vi "foobar.vi"(8 "error in (no error)":errorcluster, 11 "Model in":refnum<class "Model.lvclass">) -> (0 "error out":errorcluster, 3 "Model out":refnum<class "Model.lvclass">)   [LabVIEW 2016, in "Model.lvclass"]
uses:
  Model.lvclass
  Model.lvclass/Model.ctl
  ILCCommunications/ILCCommunications.lvclass
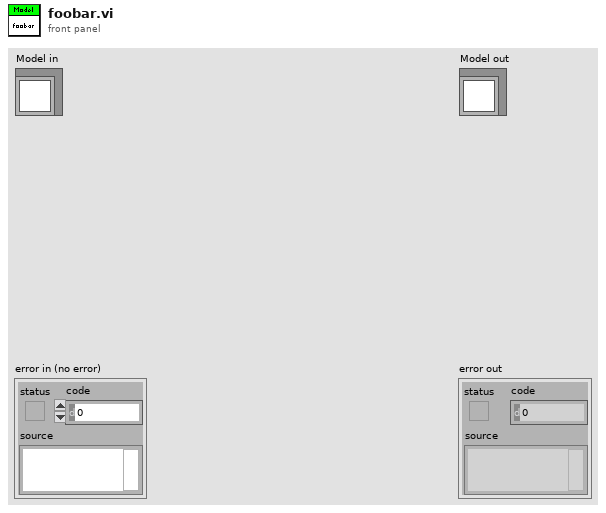
[diagram p1: front panel]
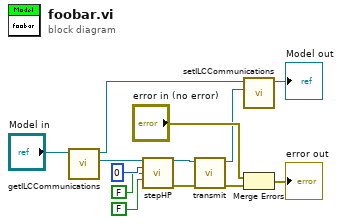
[diagram p0: block diagram]
diagram:
  n1 = call "getILCCommunications.vi"("Model in"="Model in") -> ("ILCCommunications"=w10:refnum<class "ILCCommunications.lvclass">, "Model out"=w4:refnum<class "Model.lvclass">)  [unwired: 9 in]
  n2 = call "stepHP.vi"("ILCCommunications in"=w10, "HPIndex"=0, "WaitForTrigger"=FALSE, "TriggerIRQ"=FALSE) -> ("ILCCommunications out"=w6:refnum<class "ILCCommunications.lvclass">, "error out"=w5:errorcluster)  [unwired: 10 in]
  n3 = call "transmit.vi"("error in (no error)"=w5, "ILCCommunications in"=w6) -> ("error out"=w1:errorcluster, "ILCCommunications out"=w3:refnum<class "ILCCommunications.lvclass">)  [unwired: 8 in]
  n4 = call "setILCCommunications.vi"("ILCCommunications"=w3, "Model in"=w4) -> ("Model out"=→"Model out":refnum<class "Model.lvclass">)  [unwired: 9 in]
  n5 = Merge Errors("error in (no error)", w1) -> (→"error out":errorcluster)
